vi "Time Delay - Variable mS.vi"(1 "milliseconds to wait":u32, 3 "error in (no error)":errorcluster) -> (0 "error out":errorcluster)   [LabVIEW 2018]
doc: "Inserts a delay of a specified length in milliseconds. By wiring to error in and error out, it is easy to force a delay at a desired point in a sequence of operations.\n\nIf no error in: wait <delay> ms then continue\n\nIf error in: do not delay - pass error out"
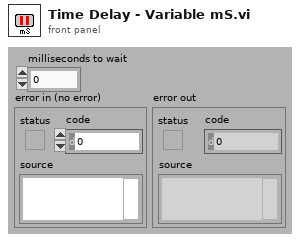
[diagram p1: front panel]
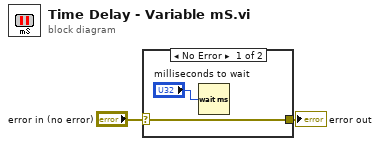
[diagram p0: block diagram]
diagram:
  n1 = case shown="No Error" "error in (no error)" {
    selector: "error in (no error)" -> [w4 w5]
    tunnel: [w4 w5] -> w1
    frame No Error {
      n2 = Wait (ms)(milliseconds to wait="milliseconds to wait") -> ()  [unwired: 1 out]
    }
    frame Error {
    }
  }
  "error out" <- w1
